vi "Parse Limit Switch Position.vi"(11 "QS Response":string) -> (2 "At Switch?":bool, 3 "motor":i32)   [LabVIEW 2024, in "FW Arduino Control.lvclass"]
uses:
  FW Arduino Control.lvclass
  <vilib>/regexp/Match Regular Expression.xnode
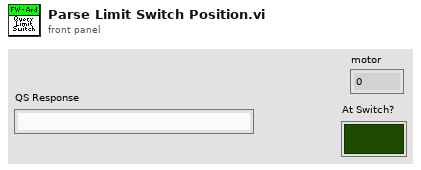
[diagram p1: front panel]
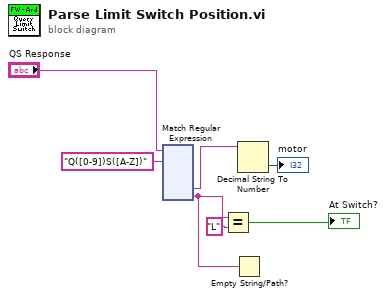
[diagram p0: block diagram]
diagram:
  n1 = xnode "Match Regular Expression"("input string"="QS Response", "regular expression"="Q([0-9])S([A-Z])") -> ("submatch 1"=w5:string, "submatch 2"=w1:string)  [unwired: 4 in, 5 out]
  n2 = Equal?(x=w1, y="L") -> (x = y?=→"At Switch?":bool)
  n3 = Empty String/Path?(string/path=w1) -> ()  [unwired: 1 out]
  n4 = Decimal String To Number(string=w5) -> (number=→"motor":i32)  [unwired: 2 in, 1 out]
